vi "EE_DataLoggingLoopTXT.vi"(6 "StopButton Refnum":refnum<vi>, 8 "EEG Record Refnum":refnum<vi>, 9 "UserName":string, 10 "Logs directory path":path, 11 "ChannelsDataNotifier in":T2) -> (3 "ChannelsDataNotifier out":T2)   [LabVIEW 2016, in "Emotiv Epoc.lvlib"]
uses:
  EE_Notifier_Refnum.ctl
  EE_Notifier_Data_Type.ctl
  EE_SignalStrength_enum.ctl
  EE_EEG_ContactQuality_enum.ctl
  Emotiv_EEG_Channels_enum.ctl
  <vilib>/Utility/file.llb/Write Delimited Spreadsheet (string).vi
  <vilib>/Utility/file.llb/Write Delimited Spreadsheet (DBL).vi
  Emotiv Epoc.lvlib
  EmotivEpocHeadsetControls.lvclass
panel:
  in  "Emotiv_EEG_Channels_enum":T1
  # "This VI is a part of BCI Design library, http://www.ru-bci.org \nCopyright © 2020, Sotnikov Peter, All rights reserved. License: GNU GPLv3"
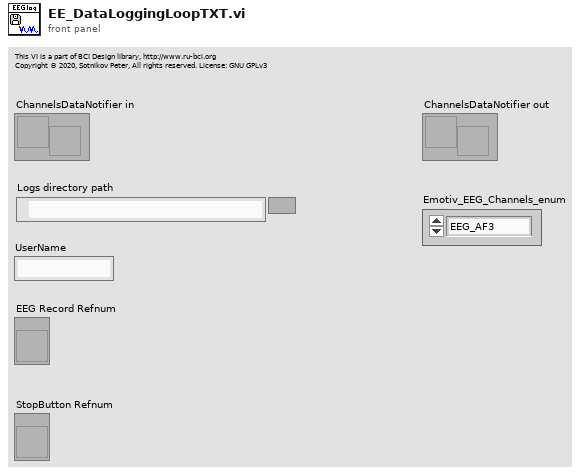
[diagram p1: front panel]
types:
  T1 = typedef "Emotiv Epoc.lvlib/Emotiv_EEG_Channels_enum.ctl" = enum16{"EEG_AF3", "EEG_F7", "EEG_F3", "EEG_FC5", "EEG_T7", "EEG_P7", "EEG_O1", "EEG_O2", "EEG_P8", "EEG_T8", "EEG_FC6", "EEG_F4", "EEG_F8", "EEG_AF4"}
  T2 = typedef "Emotiv Epoc.lvlib/EE_Notifier_Refnum.ctl" = refnum<notifier>
  T3 = typedef "Emotiv Epoc.lvlib/EE_Notifier_Data_Type.ctl" = cluster{"EDK_Error":string, "Number of samples":u32, "Marker Waveform":waveform(dbl), "Array of EEG waveforms":waveform(dbl)[], "WirelessSignalStatus":T4, "EEG_ContactsQuality":T5[]}
  T4 = typedef "Emotiv Epoc.lvlib/EmotivEpocHeadsetControls.lvclass/EE_SignalStrength_enum.ctl" = enum32{"NO_SIGNAL", "BAD_SIGNAL", "GOOD_SIGNAL"}
  T5 = typedef "Emotiv Epoc.lvlib/EE_EEG_ContactQuality_enum.ctl" = enum16{"EEG_CQ_NO_SIGNAL", "EEG_CQ_VERY_BAD", "EEG_CQ_POOR", "EEG_CQ_FAIR", "EEG_CQ_GOOD"}
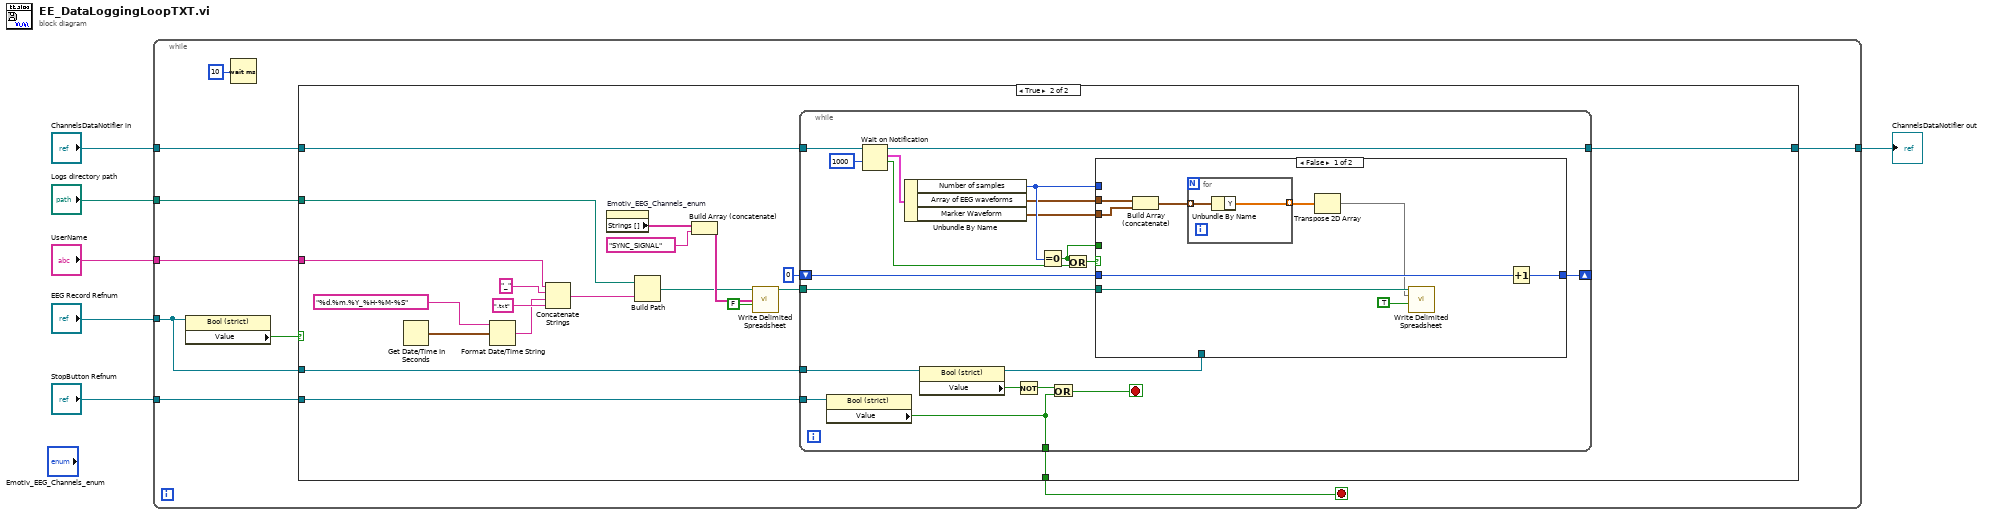
[diagram p0: block diagram]
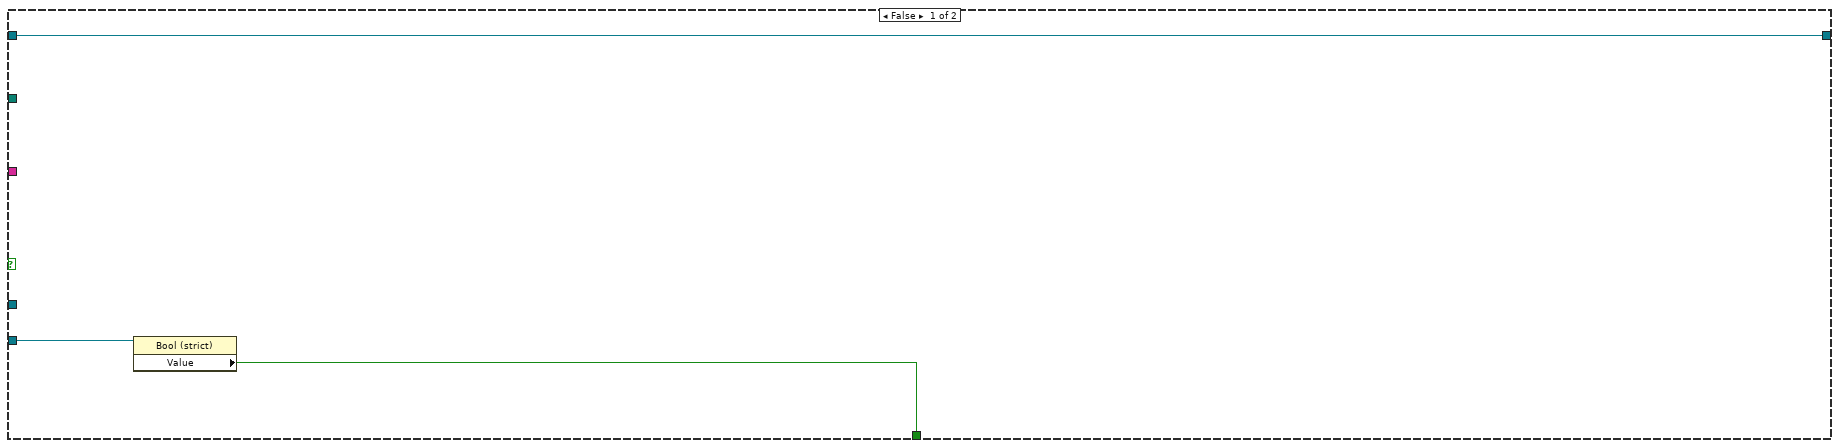
[diagram p2: hidden frame]
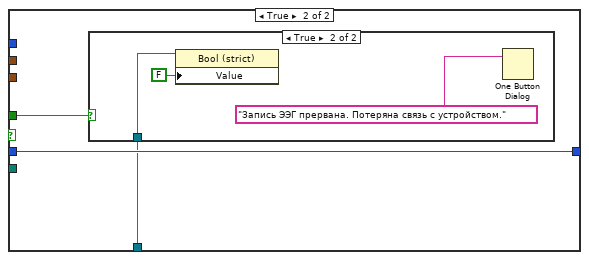
[diagram p3: hidden frame]
diagram:
  n1 = while {
    tunnel: "EEG Record Refnum" -> [w10]
    tunnel: "UserName" -> [w14]
    tunnel: "Logs directory path" -> [w13]
    tunnel: "ChannelsDataNotifier in" -> [w12]
    tunnel: [w11] -> w1
    tunnel: "StopButton Refnum" -> [w9]
    stop <- w8 stop-if-true
    n2 = property class="Bool (strict)"(reference=w10) -> ("Value"=w15:bool)  [unwired: 1 in, 2 out]
    n3 = Wait (ms)(milliseconds to wait=u32 10) -> ()  [unwired: 1 out]
    n4 = case shown="True" w15 {
      tunnel: w14 -> [_ w33]
      tunnel: w13 -> [_ w32]
      tunnel: w12 -> [w18 w31]
      tunnel: [w18 w30] -> w11
      tunnel: w10 -> [_ w29]
      tunnel: w9 -> [w17 w28]
      tunnel: [w16 w27] -> w8
      frame False {
        n5 = property class="Bool (strict)"(reference=w17) -> ("Value"=w16:bool)  [unwired: 1 in, 2 out]
      }
      frame True {
        n6 = Get Date/Time In Seconds() -> (seconds since 1Jan1904=w34:timestamp)
        n7 = Format Date/Time String(time format string (%c)="%d.%m.%Y_%H-%M-%S", seconds (now)=w34) -> (date/time string=w36:string)  [unwired: 1 in]
        n8 = Concatenate Strings(w33, "_" ("string"), w36, ".txt" ("string")) -> (w25:string)
        n9 = property on="Emotiv_EEG_Channels_enum" class="Enum (strict)"() -> ("Strings []"=w24:string[])  [unwired: 2 in, 2 out]
        n10 = Build Path(base path=w32, name or relative path=w25) -> (appended path=w21:path)
        n11 = Build Array (concatenate)(w24, "SYNC_SIGNAL") -> (w22:string[])
        n12 = call-poly <vilib>:"Write Delimited Spreadsheet.vi"("file path (dialog if empty)"=w21, "1D data"=w22, "append to file? (new file:F)"=FALSE) -> ("new file path (Not A Path if cancelled)"=w20:path)  [unwired: 11 in, 1 out]
        n13 = while {
          tunnel: w20 -> [w58]
          tunnel: w31 -> [w57]
          tunnel: [w55] -> w30
          tunnel: w29 -> [w54]
          tunnel: w28 -> [w53]
          tunnel: [w49] -> w27
          shift-right: [w47] -> _
          shift-left: 0 -> [w48]
          stop <- w50 stop-if-true
          n14 = property class="Bool (strict)"(reference=w53) -> ("Value"=w49:bool)  [unwired: 1 in, 2 out]
          n15 = Wait on Notification(notifier=w57, timeout in ms (-1)=1000) -> (notifier out=w55:T2, notification=w46:T3, timed out?=w44:bool)  [unwired: 2 in, 1 out]
          n16 = Unbundle By Name(w46) -> ("Number of samples"=w43:u32, "Array of EEG waveforms"=w42:waveform(dbl)[], "Marker Waveform"=w41:waveform(dbl))
          n17 = property class="Bool (strict)"(reference=w54) -> (reference out=w39:refnum<vi>, "Value"=w52:bool)  [unwired: 1 in, 1 out]
          n18 = Not(x=w52) -> (.not. x?=w51:bool)
          n19 = Equal To 0?(x=w43) -> (x = 0?=w40:bool)
          n20 = Or(x=w51, y=w49) -> (x .or. y?=w50:bool)
          n21 = Or(x=w40, y=w44) -> (x .or. y?=w45:bool)
          n22 = case shown="False" w45 {
            tunnel: w58 -> [w62 _]
            tunnel: w48 -> [w67 w72]
            tunnel: [w66 w72] -> w47
            tunnel: w43 -> [_ _]
            tunnel: w42 -> [w65 _]
            tunnel: w41 -> [w64 _]
            tunnel: w40 -> [_ w71]
            tunnel: w39 -> [_ w70]
            frame False {
              n23 = Build Array (concatenate)(w65, w64) -> (w63:waveform(dbl)[])
              n24 = for {
                tunnel: w63 -> [w69] mode=indexing
                tunnel: [w68] -> w61 mode=indexing
                n25 = Unbundle By Name(w69) -> ("Y"=w68:dbl[])
              }
              n26 = Transpose 2D Array(2D array=w61) -> (transposed array=w60:dbl[][])
              n27 = call-poly <vilib>:"Write Delimited Spreadsheet.vi"("file path (dialog if empty)"=w62, "2D data"=w60, "append to file? (new file:F)"=TRUE) -> ()  [unwired: 11 in, 2 out]
              n28 = Increment(x=w67) -> (x+1=w66:i32)
            }
            frame True {
              n29 = case shown="True" w71 {
                tunnel: w70 -> [_ w75]
                frame False {
                }
                frame True {
                  n30 = property class="Bool (strict)"(reference=w75, "Value"=FALSE) -> ()  [unwired: 1 in, 2 out]
                  n31 = One Button Dialog(message="Запись ЭЭГ прервана. Потеряна связь с устройством.") -> ()  [unwired: 1 in, 1 out]
                }
              }
            }
          }
        }
      }
    }
  }
  "ChannelsDataNotifier out" <- w1
